vi "Check if Path Is Test Class.vi"(8 "error in":errorcluster, 11 "Test Class Path":path) -> (0 "error out":errorcluster, 1 "TestType":string, 2 "IsTestObject":bool)   [LabVIEW 2019, in "VITesterUtilities.lvlib"]
uses:
  Libraries/VITesterUtilities.lvlib
  JKI Reuse/X in Y (Variant)__jki_lib_array -- VI Tester.vi
  <userlib>/_OpenG.lib/file/file.llb/Strip Path Extension - String__ogtk.vi
  JKI Reuse/Filter Error Codes (Scalar)__jki_lib_error_handling -- VI Tester.vi
  Classes/TestCase/TestCase.lvclass
  Classes/TestSuite/TestSuite.lvclass
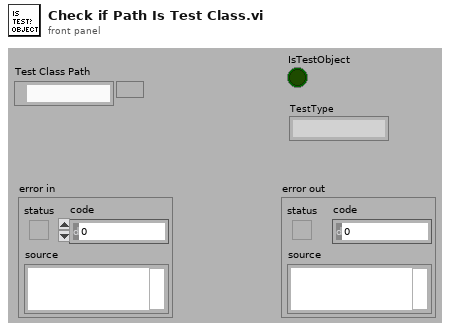
[diagram p1: front panel]
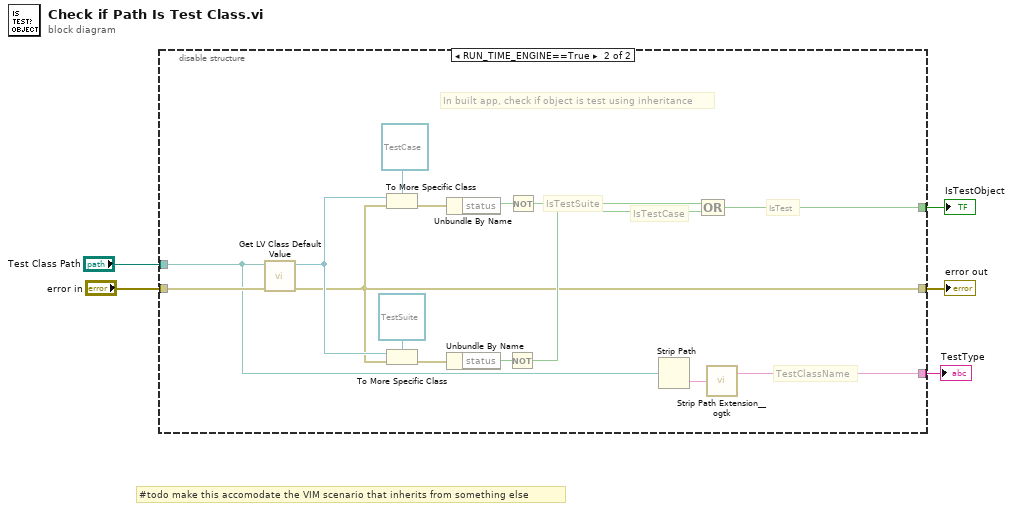
[diagram p0: block diagram]
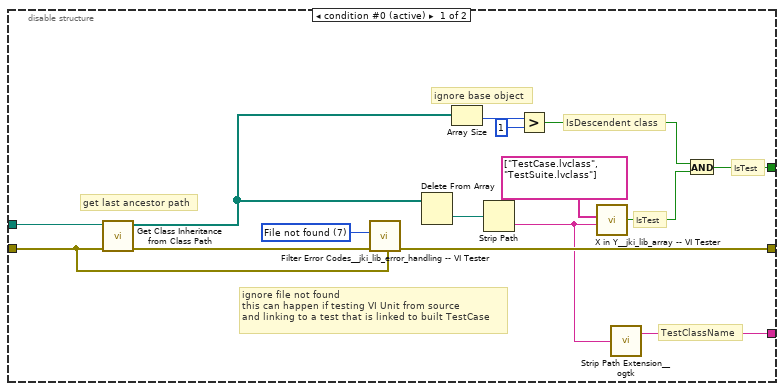
[diagram p2: hidden frame]
diagram:
  # "#todo make this accomodate the VIM scenario that inherits from something else"
  n1 = disable-structure shown="RUN_TIME_ENGINE==True" {
    disable-tunnel: [w20 w24] -> w5
    disable-tunnel: "Test Class Path" -> [w19 w25]
    disable-tunnel: "error in" -> [w18 w26]
    disable-tunnel: [w17 w23] -> w2
    disable-tunnel: [w16 w22] -> w1
    frame condition #0 (active) {
      w13 = 7 items=["No error", "Argument error", "Memory is full", "Out of zone", "End of file", "File already open", "Generic file I/O error", "File not found", "File permission error", "Disk is full", "Duplicate path", "Too many files open", "System feature not enabled", "Resource file not found", "Cannot add resource", "Resource not found", "Image not found", "Image memory error", "Pen does not exist", "Config type invalid", "Config token not found", "Config parse error", "Config memory error", "Bad external code format", "Bad external code offset", "External code not present", "Null window", "Destroy window error", "Null menu", "Print aborted", "Bad print record", "Print driver error", "Windows error during printing", "Memory error during printing", "Print dialog error", "Generic print error", "Invalid device refnum", "Device not found", "Device parameter error", "Device unit error", "Cannot open device", "Device call aborted", "Generic error", "Cancelled by user", "Object ID too low", "Object ID too high", "Object not in heap", "Unknown heap", "Unknown object (invalid DefProc)", "Unknown object (DefProc not in table)", "Message out of range", "Invalid (null) method", "Unknown message", "Manager call not supported", "Bad address", "Network operation in progress", "Network operation timed out", "Connection is busy", "Network attribute not supported", "Network error", "Address in use", "System out of memory", "Connection aborted", "Connection refused", "Not connected", "Already connected", "Connection closed", "Initialization error (interapplication manager)", "Bad occurrence", "Wait on unbound occurrence handler", "Occurrence queue overflow", "Datalog type conflict", "Unused", "Unrecognized type (interapplication manager)", "Memory corrupt", "Failed to make temporary DLL", "Old CIN version", "Drag socket not found", "Failed to load drop-object", "Failed to register OLE object", "Failed to release OLE object", "Format specifier type mismatch", "Unknown format specifier", "Too few format specifiers", "Too many format specifiers", "Scan failed", "Newer CIN version", "Error converting to variant", "Runtime menu error", "Password tampered", "Variant attribute not found", "Incompatible variant data type", "Event data is not available", "Event Store is not present", "Occurrence is not found", "Event Queue is not created", "Event info is not available", "Refnum passed is NULL", "Error retrieving Class GUID", "Error retrieving CoClass GUID", "Error retrieving TypeLib GUID.", "Bad built application magic bytes.", "Specific driver is different from the specific driver associated with the Logical Name.", "There is no session opened to the class driver.", "Max Error", "MAX - Error with config objects", "MAX - Error loading configuration", "MAX - Group not supported"]
      # "TestClassName"
      # "IsTest"
      # "IsTest"
      # "IsDescendent class"
      # "ignore base object"
      # "get last ancestor path"
      # "ignore file not found\nthis can happen if testing VI Unit from source\nand linking to a test that is linked to built TestCase"
      n2 = call "Get Class Inheritance from Class Path.vi"("error in (no error)"=w18, "lvclass file Path"=w19) -> ("error out"=w14:errorcluster, "Class Inheritance [ ]"=w12:path[])  [unwired: 8 in]
      n3 = call-poly "Filter Error Codes__jki_lib_error_handling -- VI Tester.vi"("upstream error (optional)"=w18, "error in"=w14, "error code to filter"=w13) -> ("error out"=w20:errorcluster)  [unwired: 6 in, 2 out]
      n4 = Delete From Array(array=w12) -> (deleted portion=w15:path)  [unwired: 2 in, 1 out]
      n5 = Array Size(array=w12) -> (size(s)=w11:i32)
      n6 = Strip Path(path=w15) -> (name=w6:string)  [unwired: 1 out]
      n7 = Greater?(x=w11, y=1) -> (0:w9:bool)
      n8 = call-poly "X in Y__jki_lib_array -- VI Tester.vi"("array"=string[] ["TestCase.lvclass", "TestSuite.lvclass"], "element"=w6) -> ("element in array?"=w8:bool)  [unwired: 5 in]
      n9 = call-poly <userlib>:"Strip Path Extension__ogtk.vi"("path"=w6) -> ("root"=w16:string)  [unwired: 1 out]
      n10 = And(x=w9, y=w8) -> (x .and. y?=w17:bool)
    }
    frame condition #1 {
      # "TestClassName"
      # "IsTest"
      # "IsTestSuite"
      # "IsTestCase"
      # "In built app, check if object is test using inheritance"
      n11 = call <vilib>:"Get LV Class Default Value.vi"("error in (no error)"=w26, "class path"=w25) -> ("error out"=w24:errorcluster, "object"=w28:refnum<class>)  [unwired: 8 in]
      n12 = To More Specific Class(target class=refnum<class "TestCase.lvclass"> refnum ("TestCase.lvclass"), reference=w28, error in=w24) -> (error out=w34:errorcluster)  [unwired: 1 out]
      n13 = To More Specific Class(target class=refnum<class "TestSuite.lvclass"> refnum ("TestSuite.lvclass"), reference=w28, error in=w24) -> (error out=w35:errorcluster)  [unwired: 1 out]
      n14 = Unbundle By Name(w34) -> ("status"=w32:bool)
      n15 = Unbundle By Name(w35) -> ("status"=w31:bool)
      n16 = Not(x=w31) -> (.not. x?=w29:bool)
      n17 = Not(x=w32) -> (.not. x?=w30:bool)
      n18 = Strip Path(path=w25) -> (name=w33:string)  [unwired: 1 out]
      n19 = Compound Arithmetic op=OR(w30, w29) -> (w23:bool)
      n20 = call-poly <userlib>:"Strip Path Extension__ogtk.vi"("path"=w33) -> ("root"=w22:string)  [unwired: 1 out]
    }
  }
  "IsTestObject" <- w2
  "error out" <- w5
  "TestType" <- w1
